vi "PathSearch.vi"(0 "Path":dbl[][](array[numeric]), 5 "Reint":bool, 9 "Robot X (in)":dbl, 11 "Robot Y (in)":dbl, 12 "Search Window (s)":dbl=2.0, 13 "Look-Ahead Time (s)":dbl=0.25) -> (1 "Distance from Start (in)":dbl, 3 "Distance from End (in)":dbl, 4 "Feed Back Distance Error (in)":dbl, 6 "Feed Back Pointing Angle (deg)":dbl, 8 "Feed Forward Pointing Angle (deg)":dbl, 10 "Feed Forward Velocity (in/s)":dbl, 15 "Robot Heading Goal (deg)":dbl)   [LabVIEW 2019]
doc: "This VI takes as input the robots current pose and the loaded autonomous path. The algorithm then efficiently searches the path and identifies the nearest point and the pursuit point. The the feed-forward heading, pointing direction, and velocity are output along with the error distance and and pointing direction required to return to the path. The distance along the path is also output. The Search Window can be specified in seconds - longer search windows are more robust to recovering from large deviations from the path but may cause the robot to \"jump\" ahead when following tight loops or turns. The Look-Ahead Time specifies the furthest ahead the pursuit point can be."
panel:
  out "Look-Ahead Point":i32
  out "Closest Point":i32
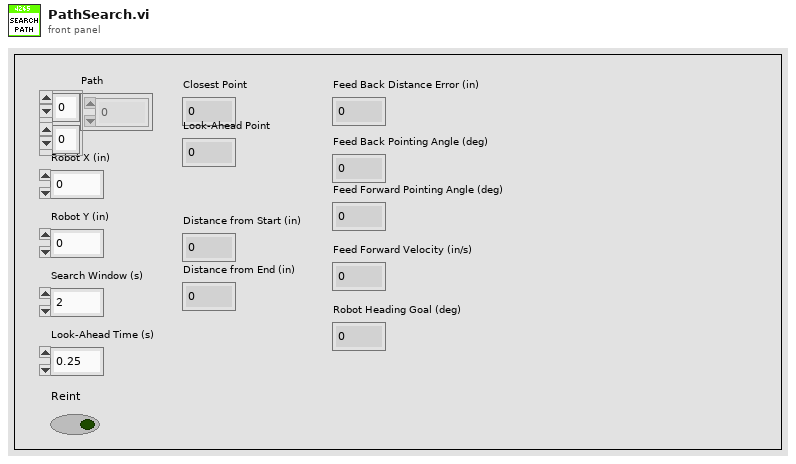
[diagram p1: front panel]
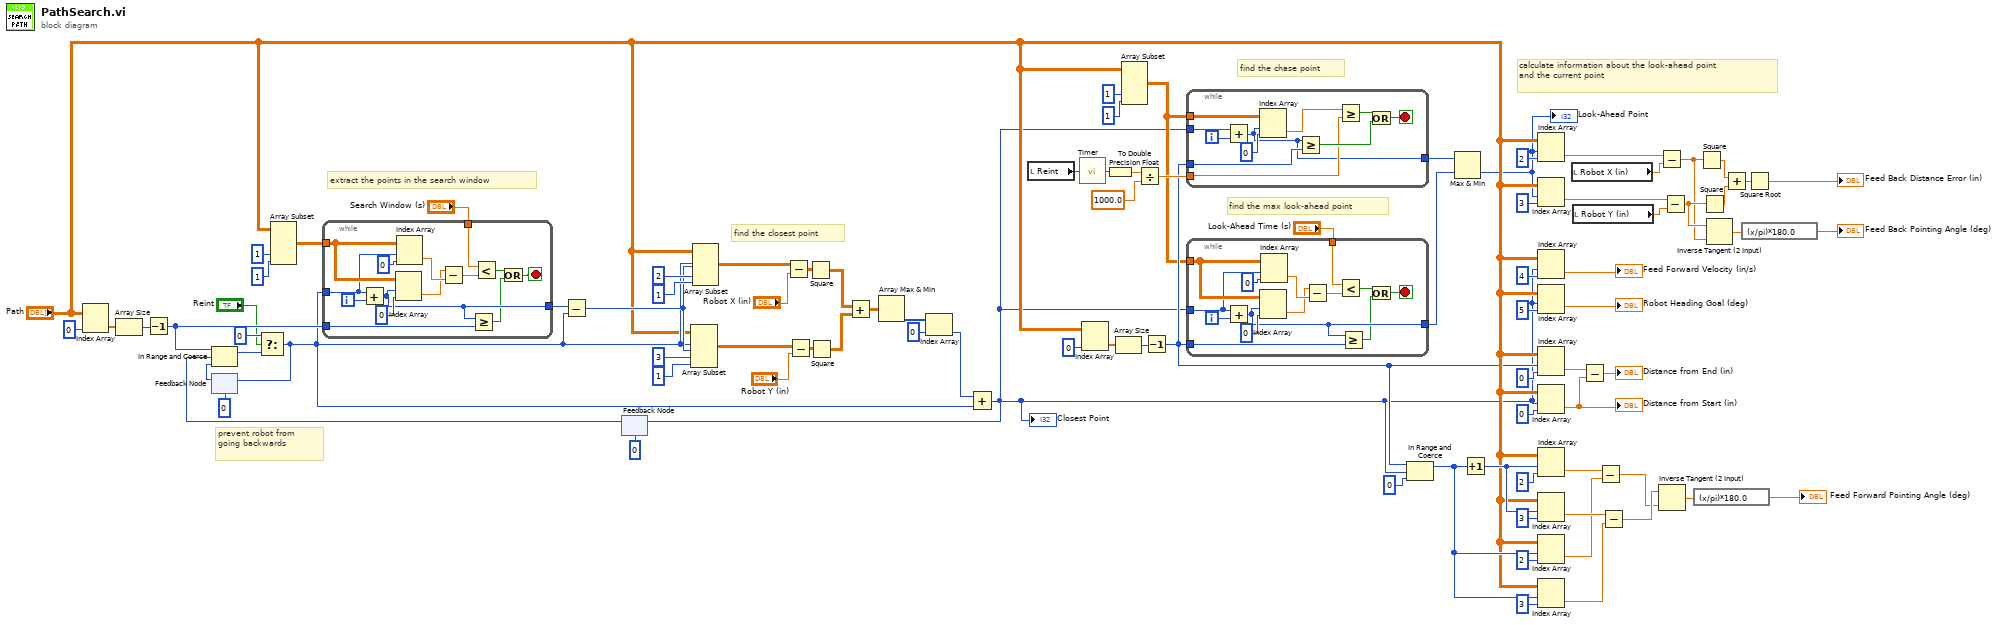
[diagram p0: block diagram]
diagram:
  # "find the chase point"
  # "find the max look-ahead point"
  # "calculate information about the look-ahead point\nand the current point"
  # "prevent robot from \ngoing backwards"
  # "find the closest point"
  # "extract the points in the search window"
  n1 = Index Array(array="Path", index (col)=0 ("disabled index (col)")) -> (element=w52:dbl[])  [unwired: 1 in]
  n2 = Array Size(array=w52) -> (size(s)=w53:i32)
  n3 = Decrement(x=w53) -> (x-1=w49:i32)
  n4 = feedback #1(0) -> (w50:i32)
  n5 = Array Subset(array="Path", index (col)=1 ("index"), length (col)=1 ("length")) -> (w73:dbl[][])  [unwired: 2 in]
  n6 = feedback #2(0) -> (w48:i32)
  n7 = In Range and Coerce(upper limit=w49, x=w48, lower limit=w50) -> (coerced(x)=w31:i32)  [unwired: 1 out]
  n8 = Select(t=0, s="Reint", f=w31) -> (s? t:f=w30:i32)
  n9 = feedback-in #1(w30) -> ()
  n10 = while {
    tunnel: w30 -> [w101]
    tunnel: w73 -> [w102]
    tunnel: "Search Window (s)" -> [w96]
    tunnel: [w95] -> w71
    tunnel: w49 -> [w91]
    i -> [w104]
    stop <- w93 stop-if-true
    # "Search window"
    n11 = Add(x=w101, y=w104) -> (x+y=w95:i32)
    n12 = Index Array(array=w102, index (row)=w95, index (col)=0 ("disabled index (col)")) -> (element=w98:dbl)
    n13 = Index Array(array=w102, index (row)=w101, index (col)=0 ("disabled index (col)")) -> (element=w99:dbl)
    n14 = Subtract(x=w98, y=w99) -> (x-y=w97:dbl)
    n15 = Greater Or Equal?(x=w95, y=w91) -> (x >= y?=w92:bool)
    n16 = Less?(x=w96, y=w97) -> (x < y?=w94:bool)
    n17 = Or(x=w94, y=w92) -> (x .or. y?=w93:bool)
  }
  n18 = Subtract(x=w71, y=w30) -> (x-y=w70:i32)
  n19 = Array Subset(array="Path", index (row)=w30, length (row)=w70, index (col)=3 ("index"), length (col)=1 ("length")) -> (w82:dbl[][])
  n20 = Array Subset(array="Path", index (row)=w30, length (row)=w70, index (col)=2 ("index"), length (col)=1 ("length")) -> (w88:dbl[][])
  n21 = Subtract(x=w88, y="Robot X (in)") -> (x-y=w87:dbl[][])
  n22 = Subtract(x=w82, y="Robot Y (in)") -> (x-y=w83:dbl[][])
  n23 = Square(x=w87) -> (x^2=w80:dbl[][])
  n24 = Square(x=w83) -> (x^2=w79:dbl[][])
  n25 = Add(x=w80, y=w79) -> (x+y=w78:dbl[][])
  n26 = Array Max & Min(array=w78) -> (min index (indices)=w77:i32[])  [unwired: 3 out]
  n27 = Index Array(array=w77, index=0) -> (element=w69:i32)
  n28 = Add(x=w69, y=w30) -> (x+y=w1:i32)
  "Closest Point" <- w1
  n29 = feedback-in #2(w1) -> ()
  n30 = local read "Reint"() -> (w11:bool)
  n31 = call "Timer.vi"("Reset Timer"=w11) -> ("Time (ms)"=w10:u32)
  n32 = Index Array(array="Path", index (col)=0 ("disabled index (col)")) -> (element=w43:dbl[])  [unwired: 1 in]
  n33 = To Double Precision Float(number=w10) -> (double precision float=w8:dbl)
  n34 = Array Size(array=w43) -> (size(s)=w37:i32)
  n35 = Array Subset(array="Path", index (col)=1 ("index"), length (col)=1 ("length")) -> (w5:dbl[][])  [unwired: 2 in]
  n36 = Divide(x=w8, y=1000.0) -> (x/y=w7:dbl)
  n37 = Decrement(x=w37) -> (x-1=w6:i32)
  n38 = while {
    tunnel: w1 -> [w112]
    tunnel: w5 -> [w113]
    tunnel: w7 -> [w106]
    tunnel: w6 -> [w108]
    tunnel: [w105] -> w4
    i -> [w115]
    stop <- w110 stop-if-true
    # "Search window"
    n39 = Add(x=w112, y=w115) -> (x+y=w105:i32)
    n40 = Index Array(array=w113, index (row)=w105, index (col)=0 ("disabled index (col)")) -> (element=w107:dbl)
    n41 = Greater Or Equal?(x=w105, y=w108) -> (x >= y?=w109:bool)
    n42 = Greater Or Equal?(x=w107, y=w106) -> (x >= y?=w111:bool)
    n43 = Or(x=w111, y=w109) -> (x .or. y?=w110:bool)
  }
  n44 = while {
    tunnel: w1 -> [w126]
    tunnel: w5 -> [w127]
    tunnel: "Look-Ahead Time (s)" -> [w121]
    tunnel: [w120] -> w3
    tunnel: w6 -> [w116]
    i -> [w129]
    stop <- w118 stop-if-true
    # "Search window"
    n45 = Add(x=w126, y=w129) -> (x+y=w120:i32)
    n46 = Index Array(array=w127, index (row)=w120, index (col)=0 ("disabled index (col)")) -> (element=w123:dbl)
    n47 = Index Array(array=w127, index (row)=w126, index (col)=0 ("disabled index (col)")) -> (element=w124:dbl)
    n48 = Subtract(x=w123, y=w124) -> (x-y=w122:dbl)
    n49 = Less?(x=w121, y=w122) -> (x < y?=w119:bool)
    n50 = Greater Or Equal?(x=w120, y=w116) -> (x >= y?=w117:bool)
    n51 = Or(x=w119, y=w117) -> (x .or. y?=w118:bool)
  }
  n52 = In Range and Coerce(upper limit=w6, x=w1, lower limit=0) -> (coerced(x)=w15:i32)  [unwired: 1 out]
  n53 = Max & Min(x=w4, y=w3) -> (min(x,y)=w2:i32)  [unwired: 1 out]
  "Look-Ahead Point" <- w2
  n54 = Increment(x=w15) -> (x+1=w24:i32)
  n55 = Index Array(array="Path", index (row)=w2, index (col)=2 ("disabled index (col)")) -> (element=w66:dbl)
  n56 = Index Array(array="Path", index (row)=w2, index (col)=3 ("disabled index (col)")) -> (element=w64:dbl)
  n57 = Index Array(array="Path", index (row)=w1, index (col)=4 ("disabled index (col)")) -> (element=→"Feed Forward Velocity (in/s)":dbl)
  n58 = Index Array(array="Path", index (row)=w1, index (col)=5 ("disabled index (col)")) -> (element=→"Robot Heading Goal (deg)":dbl)
  n59 = Index Array(array="Path", index (row)=w6, index (col)=0 ("disabled index (row)")) -> (element=w34:dbl)
  n60 = Index Array(array="Path", index (row)=w1, index (col)=0 ("disabled index (col)")) -> (element=w32:dbl)
  "Distance from Start (in)" <- w32
  n61 = Index Array(array="Path", index (row)=w24, index (col)=2 ("disabled index (col)")) -> (element=w22:dbl)
  n62 = Index Array(array="Path", index (row)=w24, index (col)=3) -> (element=w23:dbl)
  n63 = Index Array(array="Path", index (row)=w15, index (col)=2) -> (element=w19:dbl)
  n64 = Index Array(array="Path", index (row)=w15, index (col)=3) -> (element=w18:dbl)
  n65 = local read "Robot X (in)"() -> (w65:dbl)
  n66 = local read "Robot Y (in)"() -> (w63:dbl)
  n67 = Subtract(x=w34, y=w32) -> (x-y=→"Distance from End (in)":dbl)
  n68 = Subtract(x=w22, y=w19) -> (x-y=w17:dbl)
  n69 = Subtract(x=w23, y=w18) -> (x-y=w26:dbl)
  n70 = Subtract(x=w66, y=w65) -> (x-y=w57:dbl)
  n71 = Inverse Tangent (2 Input)(1:w17, 2:w26) -> (0:w14:dbl)
  n72 = Subtract(x=w64, y=w63) -> (x-y=w58:dbl)
  n73 = expression code="(x/pi)*180.0"(w14) -> (→"Feed Forward Pointing Angle (deg)":dbl)
  n74 = Square(x=w57) -> (x^2=w61:dbl)
  n75 = Square(x=w58) -> (x^2=w62:dbl)
  n76 = Inverse Tangent (2 Input)(1:w57, 2:w58) -> (0:w56:dbl)
  n77 = Add(x=w61, y=w62) -> (x+y=w60:dbl)
  n78 = expression code="(x/pi)*180.0"(w56) -> (→"Feed Back Pointing Angle (deg)":dbl)
  n79 = Square Root(x=w60) -> (sqrt(x)=→"Feed Back Distance Error (in)":dbl)
